vi "DotNET XML Signature.vi"(8 "error in (no error)":errorcluster, 10 "XML String In":string="<root>  \n    <creditcard>  \n        <number>19834209</number>  \n        <expiry>02/02/2002</expiry>  \n    </creditcard>  \n</root>") -> (0 "error out":errorcluster, 2 "Signed XML":string)   [LabVIEW 2016]
uses:
  System.Security
  System.Xml
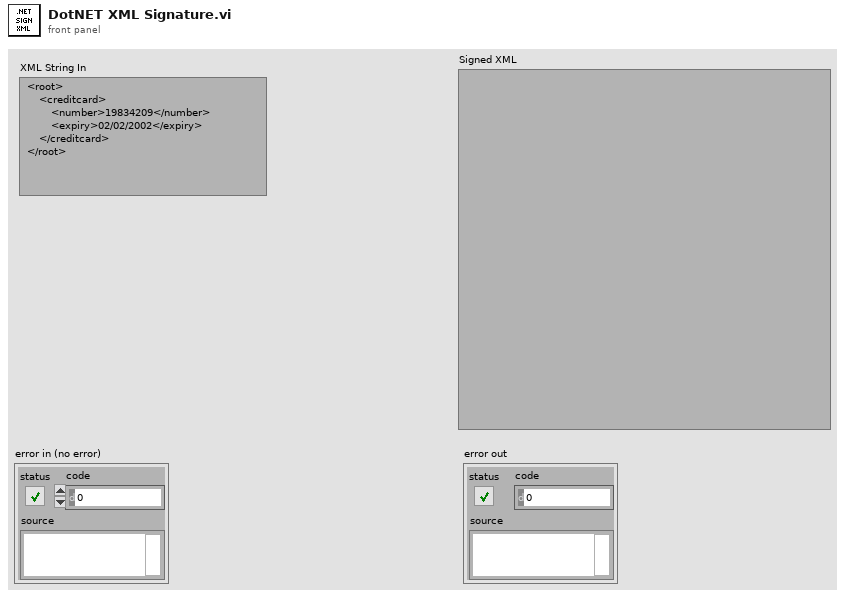
[diagram p1: front panel]
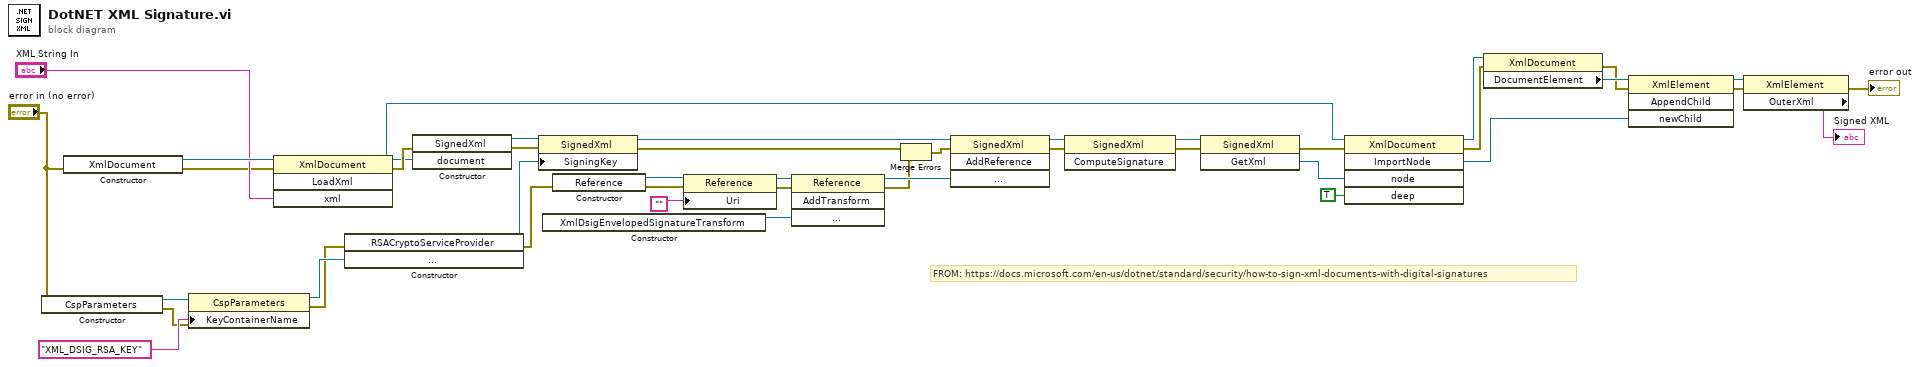
[diagram p0: block diagram]
diagram:
  # "FROM: https://docs.microsoft.com/en-us/dotnet/standard/security/how-to-sign-xml-documents-with-digital-signatures"
  n1 = constructor class="CspParameters" ("AliceErstelltPrivateKeyUndPublicKey")(error in="error in (no error)") -> (reference out=w11:refnum<k24>, error out=w8:errorcluster)  [unwired: 2 in, 1 out]
  n2 = constructor class="XmlDocument"(error in="error in (no error)") -> (reference out=w37:refnum<k24>, error out=w35:errorcluster)  [unwired: 2 in, 1 out]
  n3 = property class="CspParameters"(reference=w11, error in=w8, "KeyContainerName"="XML_DSIG_RSA_KEY") -> (reference out=w9:refnum<k24>, error out=w7:errorcluster)
  n4 = invoke class="XmlDocument" method="LoadXml"(reference=w37, error in=w35, "xml"="XML String In") -> (reference out=w23:refnum<k24>, error out=w34:errorcluster)  [unwired: 1 in, 2 out]
  n5 = constructor class="RSACryptoServiceProvider" ("AliceErstelltPrivateKeyUndPublicKey")(error in=w7, "parameters"=w9) -> (reference out=w14:refnum<k24>, error out=w6:errorcluster)  [unwired: 2 in, 2 out]
  n6 = constructor class="SignedXml"(error in=w34, "document"=w23) -> (reference out=w42:refnum<k24>, error out=w33:errorcluster)  [unwired: 2 in, 2 out]
  n7 = property class="SignedXml"(reference=w42, error in=w33, "SigningKey"=w14) -> (reference out=w39:refnum<k24>, error out=w32:errorcluster)
  n8 = constructor class="XmlDsigEnvelopedSignatureTransf"() -> (reference out=w40:refnum<k24>)  [unwired: 3 in, 2 out]
  n9 = constructor class="Reference"(error in=w6) -> (reference out=w41:refnum<k24>, error out=w5:errorcluster)  [unwired: 2 in, 1 out]
  n10 = property class="Reference"(reference=w41, error in=w5, "Uri"="") -> (reference out=w29:refnum<k24>, error out=w4:errorcluster)
  n11 = invoke class="Reference" method="AddTransform"(reference=w29, error in=w4, "transform"=w40) -> (reference out=w30:refnum<k24>, error out=w2:errorcluster)  [unwired: 1 in, 2 out]
  n12 = Merge Errors(w32, w2) -> (w3:errorcluster)
  n13 = invoke class="SignedXml" method="AddReference"(reference=w39, error in=w3, "reference"=w30) -> (reference out=w38:refnum<k24>, error out=w31:errorcluster)  [unwired: 1 in, 2 out]
  n14 = invoke class="SignedXml" method="ComputeSignature"(reference=w38, error in=w31) -> (reference out=w27:refnum<k24>, error out=w26:errorcluster)  [unwired: 1 in, 1 out]
  n15 = invoke class="SignedXml" method="GetXml"(reference=w27, error in=w26) -> (error out=w13:errorcluster, "GetXml"=w22:refnum<k24>)  [unwired: 1 in, 1 out]
  n16 = invoke class="XmlDocument" method="ImportNode"(reference=w23, error in=w13, "node"=w22, "deep"=TRUE) -> (reference out=w20:refnum<k24>, error out=w16:errorcluster, "ImportNode"=w24:refnum<k24>)  [unwired: 1 in, 2 out]
  n17 = property class="XmlDocument"(reference=w20, error in=w16) -> (error out=w15:errorcluster, "DocumentElement"=w21:refnum<k24>)  [unwired: 1 out]
  n18 = invoke class="XmlElement" method="AppendChild"(reference=w21, error in=w15, "newChild"=w24) -> (reference out=w18:refnum<k24>, error out=w12:errorcluster)  [unwired: 1 in, 2 out]
  n19 = property class="XmlElement"(reference=w18, error in=w12) -> (error out=→"error out":errorcluster, "OuterXml"=→"Signed XML":string)  [unwired: 1 out]
